vi "Tic_Tac.vi"(6 "Akcja":enum16{"Tick", "Tack"}(ring), 7 "Clear error? (T)":bool=TRUE, 11 "error in (no error)":errorcluster) -> (1 "Delay":dbl, 3 "error out":errorcluster)   [LabVIEW 2014]
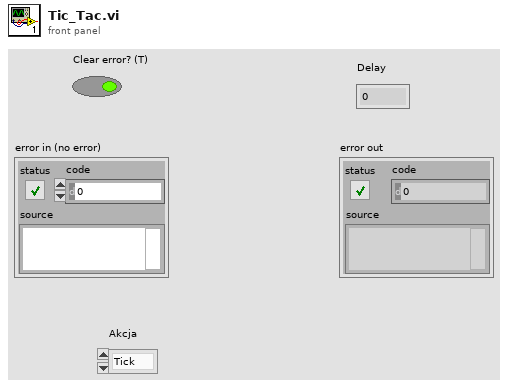
[diagram p1: front panel]
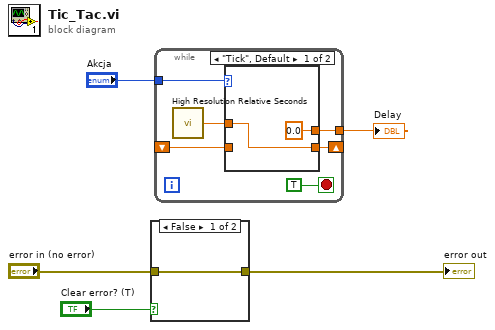
[diagram p0: block diagram]
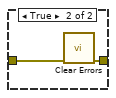
[diagram p2: hidden frame]
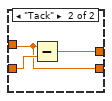
[diagram p3: hidden frame]
diagram:
  n1 = case shown="False" "Clear error? (T)" {
    tunnel: "error in (no error)" -> [w6 w8]
    tunnel: [w6 w7] -> w2
    frame False {
    }
    frame True {
      n2 = call <vilib>:"Clear Errors.vi"("error in (no error)"=w8) -> ("error out"=w7:errorcluster)  [unwired: 5 in, 1 out]
    }
  }
  "error out" <- w2
  n3 = while {
    tunnel: "Akcja" -> [w14]
    shift-right: [w11] -> _
    shift-left: _ -> [w10]
    tunnel: [w9] -> w4
    stop <- TRUE stop-if-true
    n4 = call <vilib>:"High Resolution Relative Seconds.vi"() -> ("relative seconds"=w12:dbl)
    n5 = case shown="\"Tick\", Default" w14 {
      tunnel: w12 -> [w16 w17]
      tunnel: [w16 w17] -> w11
      tunnel: w10 -> [_ w19]
      tunnel: [0.0 w18] -> w9
      frame "Tick", Default {
      }
      frame "Tack" {
        n6 = Subtract(x=w17, y=w19) -> (x-y=w18:dbl)
      }
    }
  }
  "Delay" <- w4
